vi "CSM - Generate User Global Log.vi"(6 "From Who":string, 7 "Place(\"\" to use VI's Name)":string, 8 "Error in":errorcluster caption="Error in (no error)", 10 "Arguments":string, 11 "Log":string) -> (0 "error out":errorcluster)   [LabVIEW 2020, in "Communicable State Machine.lvlib"]
doc: "<b>Inputs:</b>\n - <b>Error in</b>:\n - <b>From Who</b>:\n - <b>ModuleName</b>:\n - <b>Log</b>:\n - <b>Arguments</b>:\n\n<b>Outputs:</b>\n - <b>error out</b>:"
uses:
  Communicable State Machine.lvlib
  _CSM_GlobalLog_MSG_TYPE.ctl
  _CSM_GlobalLog_MSG.ctl
  _CSM_Response Source Message.ctl
  CSM - Make String Arguments Safe.vi
  CSM - Keywords.vi
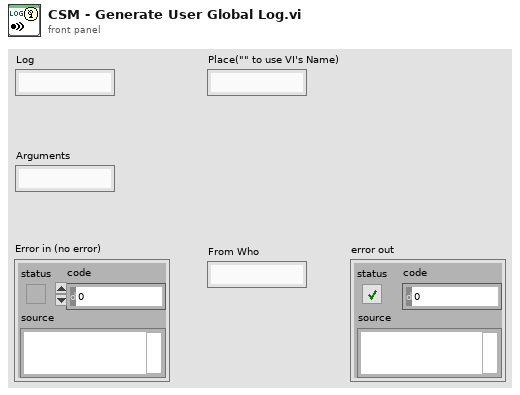
[diagram p1: front panel]
types:
  T1 = typedef "Communicable State Machine.lvlib/_CSM_GlobalLog_MSG_TYPE.ctl" = enum16{"User Log", "State Change", "Status", "Interrupt", "Register", "Unregister", "Error Log", "Module Created", "Module Destroyed"}
  T2 = typedef "Communicable State Machine.lvlib/_CSM_GlobalLog_MSG.ctl" = cluster{"Name(\"\" to use uuid)":string, "Current State":string, "Arguments":string, "Source Message":T3, "Source Module":string, "Complete(T)/Start(F)":bool, "LogType":T1}
  T3 = typedef "Communicable State Machine.lvlib/_CSM_Response Source Message.ctl" = cluster{"‘State":string, "’Arguments":string, "’Error":errorcluster}
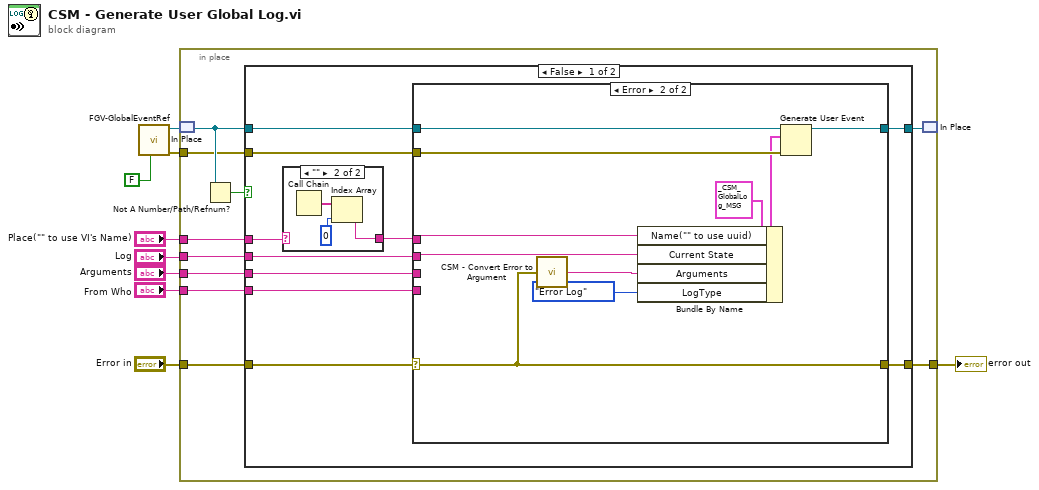
[diagram p0: block diagram]
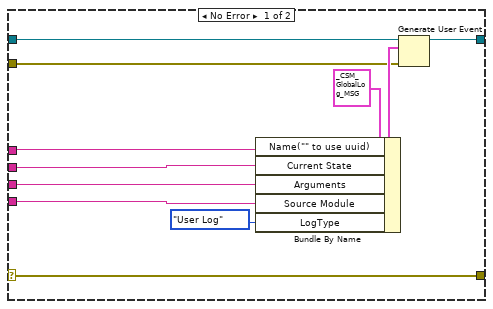
[diagram p3: hidden frame]
diagram:
  n1 = call "FGV-GlobalEventRef.vi"("Create(F)"=FALSE) -> ("error out"=w2:errorcluster, "CSM Global Log Event"=w3:refnum<user-event>)  [unwired: 9 in]
  n2 = in-place {
    in-place-border: "Place(\"\" to use VI's Name)" -> [w16]
    in-place-border: "Log" -> [w15]
    in-place-border: "Arguments" -> [w14]
    in-place-border: w2 -> [w13]
    in-place-border: [w12] -> w9
    in-place-border: "From Who" -> [w11]
    in-place-border: "Error in" -> [w10]
    n3 = in-place-match #1(w3) -> (w18:refnum<user-event>)
    n4 = Not A Number/Path/Refnum?(number/path/refnum=w18) -> (NaN/Path/Refnum?=w19:bool)
    n5 = case shown="False" w19 {
      tunnel: w18 -> [w29 w56]
      tunnel: w16 -> [w21 _]
      tunnel: [w28 w56] -> w17
      tunnel: w15 -> [w27 _]
      tunnel: w14 -> [w26 _]
      tunnel: w13 -> [w25 w55]
      tunnel: [w24 w55] -> w12
      tunnel: w11 -> [w23 _]
      tunnel: w10 -> [w22 _]
      frame False {
        n6 = case shown="\"\"" w21 {
          selector: w21 -> [w30 _]
          tunnel: [w30 w31] -> w20
          frame Default {
          }
          frame "" {
            n7 = Call Chain() -> (call chain=w32:string[])
            n8 = Index Array(array=w32, index=0 ("Index")) -> (element=w31:string)
          }
        }
        n9 = case shown="Error" w22 {
          selector: w22 -> [w35 w51]
          tunnel: w29 -> [w44 w54]
          tunnel: [w41 w52] -> w28
          tunnel: w27 -> [w40 w46]
          tunnel: w26 -> [w39 _]
          tunnel: w25 -> [w38 w53]
          tunnel: [w35 w51] -> w24
          tunnel: w23 -> [w36 _]
          tunnel: w20 -> [w34 w45]
          frame No Error {
            n10 = Bundle By Name(cluster=T2 {"Name(\"\" to use uuid)"="", "Current State"="", "Arguments"="", "Source Message"={"‘State"="", "’Arguments"="", "’Error"={"status"=FALSE, "code"=0, "source"=""}}, "Source Module"="", "Complete(T)/Start(F)"=FALSE, "LogType"=enum."User Log"} ("event data"), "Name(\"\" to use uuid)"=w34, "Current State"=w40, "Arguments"=w39, "Source Module"=w36, "LogType"=_CSM_GlobalLog_MSG_TYPE."User Log" ("Type")) -> (w42:T2)
            n11 = Generate User Event(user event=w44, event data cluster=w42, error in=w38) -> (user event out=w41:refnum<user-event>)  [unwired: 1 in, 1 out]
          }
          frame Error {
            n12 = call "CSM - Convert Error to Argument.vi"("error in (no error)"=w51) -> ("Arguments"=w47:string)  [unwired: 4 in]
            n13 = Bundle By Name(cluster=T2 {"Name(\"\" to use uuid)"="", "Current State"="", "Arguments"="", "Source Message"={"‘State"="", "’Arguments"="", "’Error"={"status"=FALSE, "code"=0, "source"=""}}, "Source Module"="", "Complete(T)/Start(F)"=FALSE, "LogType"=enum."User Log"} ("event data"), "Name(\"\" to use uuid)"=w45, "Current State"=w46, "Arguments"=w47, "LogType"=_CSM_GlobalLog_MSG_TYPE."Error Log" ("Type")) -> (w49:T2)
            n14 = Generate User Event(user event=w54, event data cluster=w49, error in=w53) -> (user event out=w52:refnum<user-event>)  [unwired: 1 in, 1 out]
          }
        }
      }
      frame True {
      }
    }
    n15 = in-place-match #1(w17) -> ()  [unwired: 1 out]
  }
  "error out" <- w9
